vi "Timestamp to DATE-DT Byte Stream.vi"(8 "error in (no error)":errorcluster, 10 "Value":timestamp) -> (0 "error out":errorcluster, 2 "Byte Stream":u8[](array[numeric]))   [LabVIEW 2018, in "TwinCAT ADS.lvclass"]
uses:
  TwinCAT ADS.lvclass
  TwinCAT.Ads
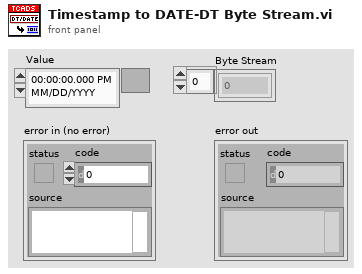
[diagram p1: front panel]
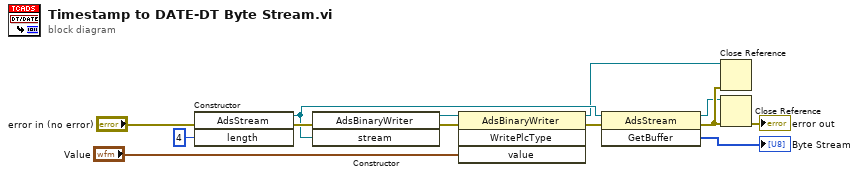
[diagram p0: block diagram]
diagram:
  n1 = constructor class="AdsStream"(error in="error in (no error)", "length"=4) -> (reference out=w9:refnum<k24>, error out=w11:errorcluster)  [unwired: 2 in, 2 out]
  n2 = constructor class="AdsBinaryWriter"(error in=w11, "stream"=w9) -> (reference out=w13:refnum<k24>, error out=w12:errorcluster)  [unwired: 2 in, 2 out]
  n3 = invoke class="AdsBinaryWriter" method="WritePlcType"(reference=w13, error in=w12, "value"="Value") -> (reference out=w6:refnum<k24>, error out=w10:errorcluster)  [unwired: 1 in, 2 out]
  n4 = invoke class="AdsStream" method="GetBuffer"(reference=w9, error in=w10) -> (reference out=w7:refnum<k24>, error out=w8:errorcluster, "GetBuffer"=→"Byte Stream":u8[])  [unwired: 1 in]
  n5 = Close Reference(reference=w6, error in (no error)=w8) -> ()  [unwired: 1 out]
  n6 = Close Reference(reference=w7, error in (no error)=w8) -> (error out=→"error out":errorcluster)
